vi "open.vi"(8 "error in (no error)":errorcluster caption="错误输入（无错误）", 11 "THM-V6数字型温湿度 输入":refnum<class "THM-V6数字型温湿度.lvclass">) -> (0 "error out":errorcluster caption="错误输出", 3 "THM-V6数字型温湿度 输出":refnum<class "THM-V6数字型温湿度.lvclass">)   [LabVIEW 2016, in "THM-V6数字型温湿度.lvlib" / "THM-V6数字型温湿度.lvclass"]
uses:
  <vilib>/Plasmionique/MB Master/MB_Master_Serial/MB_Master_Serial.lvclass
  C:/Program Files (x86)/National Instruments/LabVIEW 2016/vi.lib/Plasmionique/MB Master/MB_Master/MB_Master.lvclass
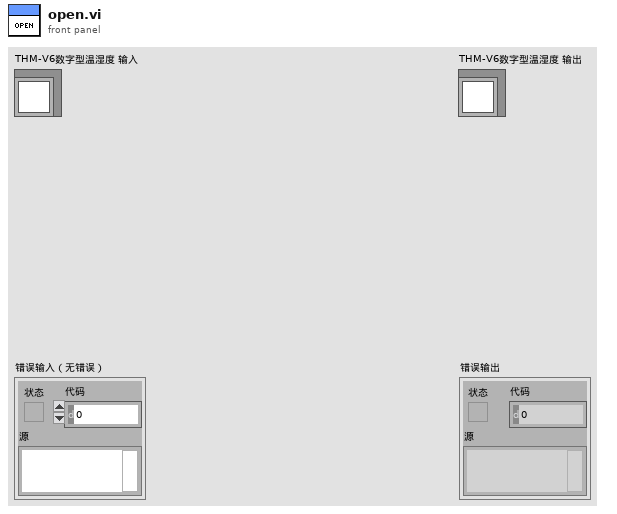
[diagram p1: front panel]
types:
  T1 = cluster{"baud rate (bps)":u32, "stop bits":u16, "parity":u16, "flow control":u16, "timeout":u32, "retries":i32}
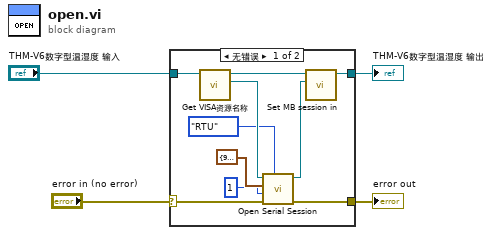
[diagram p0: block diagram]
diagram:
  n1 = case shown="无错误" "error in (no error)" {
    selector: "error in (no error)" -> [w7 w16]
    tunnel: [w5 w16] -> w3
    tunnel: [w6 w15] -> w1
    tunnel: "THM-V6数字型温湿度 输入" -> [w14 w15]
    frame No Error {
      n2 = call "Get VISA资源名称.vi"("THM-V6数字型温湿度 in"=w14) -> ("VISA资源名称"=w13:refnum<visa-resource-name>, "THM-V6数字型温湿度 out"=w8:refnum<class "THM-V6数字型温湿度.lvclass">)  [unwired: 9 in]
      n3 = call <vilib>:"Open Serial Session.vi"("Mode (RTU)"=enum16{"RTU", "ASCII"}."RTU", "Error in"=w7, "Slave ID"=u8 1, "Serial Config"=T1 {"baud rate (bps)"=9600, "stop bits"=10, "parity"=0, "flow control"=0, "timeout"=1000, "retries"=1}, "VISA Resource"=w13) -> ("Error out"=w5:errorcluster, "MB_Serial session"=w9:refnum<class "MB_Master_Serial.lvclass">)  [unwired: 5 in]
      n4 = call "Set MB session in.vi"("MB Serial Master:MB_Master"=w9, "THM-V6数字型温湿度 in"=w8) -> ("THM-V6数字型温湿度 out"=w6:refnum<class "THM-V6数字型温湿度.lvclass">)  [unwired: 9 in]
    }
    frame Error {
    }
  }
  "error out" <- w3
  "THM-V6数字型温湿度 输出" <- w1
